vi "Refr_index_to_Tvi.vi"(9 "refr inx":dbl=53.0) -> (1 "Out of  Range":bool, 3 "T tune to":dbl=97.72219547120214)   [LabVIEW 2010]
uses:
  <vilib>/gmath/NI_Gmath.lvlib
panel:
  out "refr inx out":dbl=53.0
  out "Temperature vs refractive index":cluster{"Refr index raw":dbl[], "yi":dbl[]}[](graph)=[{"Refr index raw"=[3.51113, 3.51123, 3.51146, 3.51181, 3.51229, 3.51288, 3.51358, 3.51439, 3.51979, 3.52703, 3.53555, 3.54394], "yi"=[30.0, 40.0, 50.0, 60.0, 70.0, 80.0, 90.0, 100.0, 150.0, 200.0, 250.0, 295.0]}, {"Refr index raw"=[3.514190063648601], "yi"=[97.72219547120214]}]
  in  "method":i32(ring)=3 items=["nearest", "linear", "spline", "cubic Hermite", "Lagrange"]
  out "temperature":dbl[](array[numeric])=[97.72219547120214]
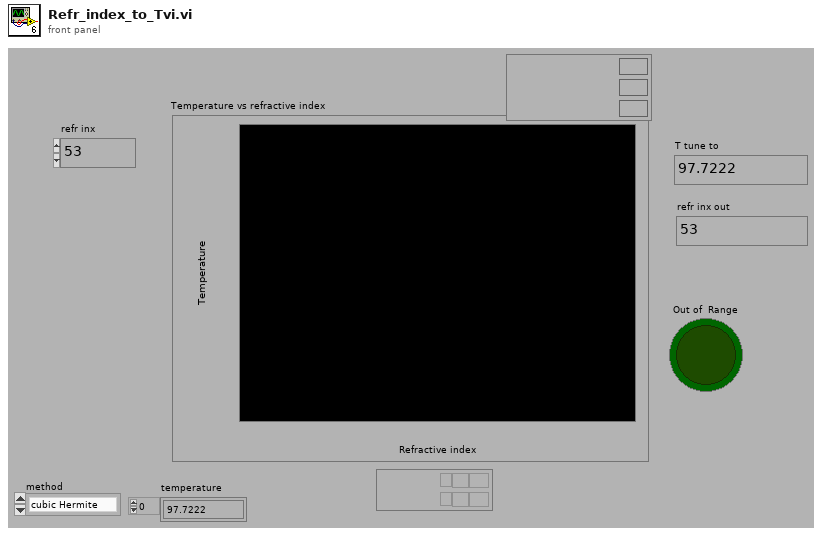
[diagram p1: front panel]
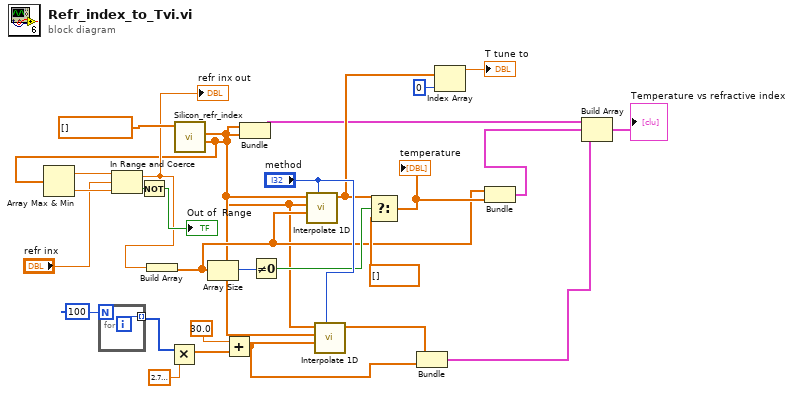
[diagram p0: block diagram]
diagram:
  n1 = for {
    N: 100 -> [_]
    tunnel: [w30] -> w27 mode=indexing
    i -> [w30]
  }
  n2 = Multiply(x=w27, y=sgl 2.7) -> (x*y=w25:sgl[])
  n3 = call "Silicon_refr_index.vi"("Temperature"=dbl[] []) -> ("Refr index raw"=w3:dbl[], "T raw"=w4:dbl[])  [unwired: 8 in, 1 out]
  n4 = Array Max & Min(array=w3) -> (max value=w10:dbl, min value=w9:dbl)  [unwired: 2 out]
  n5 = In Range and Coerce(upper limit=w10, x="refr inx", lower limit=w9) -> (coerced(x)=w6:dbl, In Range?=w11:bool)
  "refr inx out" <- w6
  n6 = Not(x=w11) -> (.not. x?=→"Out of  Range":bool)
  n7 = Build Array(w6) -> (w13:dbl[])
  n8 = Array Size(array=w13) -> (size(s)=w21:i32)
  n9 = Add(x=sgl 30.0, y=w25) -> (x+y=w2:sgl[])
  n10 = Bundle("Refr index raw"=w3, "T raw"=w4) -> (w16:cluster{"Refr index raw":dbl[], "T raw":dbl[]})  [unwired: 1 in]
  n11 = Not Equal To 0?(x=w21) -> (x != 0?=w20:bool)
  n12 = call <vilib>:"Interpolate 1D.vi"("method"="method", "xi"=w13, "X"=w3, "Y"=w4) -> ("yi"=w18:dbl[])  [unwired: 5 in, 2 out]
  n13 = call <vilib>:"Interpolate 1D.vi"("method"="method", "xi"=w2, "X"=w4, "Y"=w3) -> ("yi"=w1:dbl[])  [unwired: 5 in, 2 out]
  n14 = Select(t=w18, s=w20, f=dbl[] []) -> (s? t:f=w22:dbl[])
  "temperature" <- w22
  n15 = Bundle("yi"=w1, w2) -> (w5:cluster{"yi":dbl[], sgl[]})  [unwired: 1 in]
  n16 = Index Array(array=w18, index=0) -> (element=→"T tune to":dbl)
  n17 = Bundle(w13, "f"=w22) -> (w15:cluster{dbl[], "f":dbl[]})  [unwired: 1 in]
  n18 = Build Array(w16, w15, w5) -> (→"Temperature vs refractive index":cluster{"yi":dbl[], "f":dbl[]}[])
